vi "MSEncoder SubVI WfmCodeAccess PhaseScanII.vi"(6 "beta":ext, 8 "error in":errorcluster, 9 "Data in":T1, 11 "MSEncoder in":refnum<class "MSEncoder.lvclass">) -> (0 "error out":errorcluster, 1 "Scan time":dbl, 2 "mzTable":cluster{"t":dbl[], "mz":dbl[], "beta":dbl[]}, 3 "MSEncoder out":refnum<class "MSEncoder.lvclass">)   [LabVIEW 2018, in "MSEncoder.lvclass"]
uses:
  MSEncoder.lvclass
  MSEncoder.lvclass/MSEncoder.ctl
  WfmDataAccessor/WfmDataAccessor.lvclass
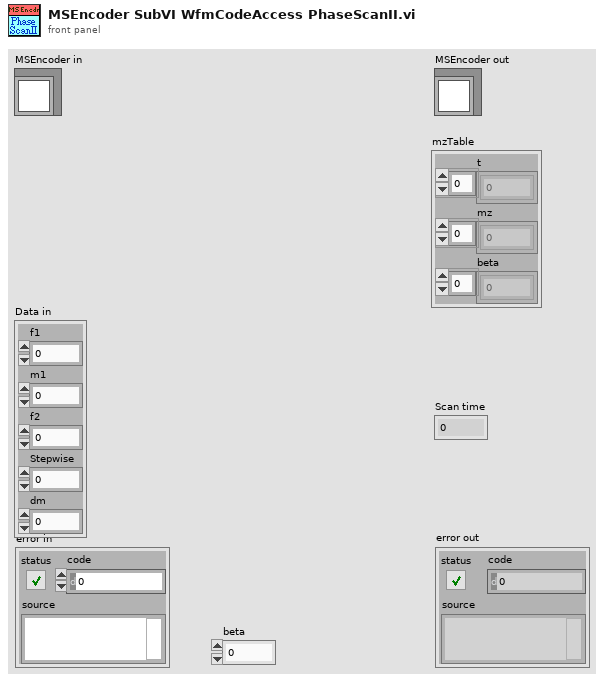
[diagram p1: front panel]
types:
  T1 = cluster{"f1":ext, "m1":ext, "f2":ext, "Stepwise":u32, "dm":ext}
  T2 = cluster{"Data in":cluster{"f1":ext, "m1":ext, "f2":ext, "Stepwise":u32, "dm":ext}, "CycDiff":u64[], "Ratio":u16[], "1/Decyc":u32, "Decyc":u32, string}
  T3 = cluster{"1/Decyc":u32, "Decyc":u64, "Actual Freq":dbl}
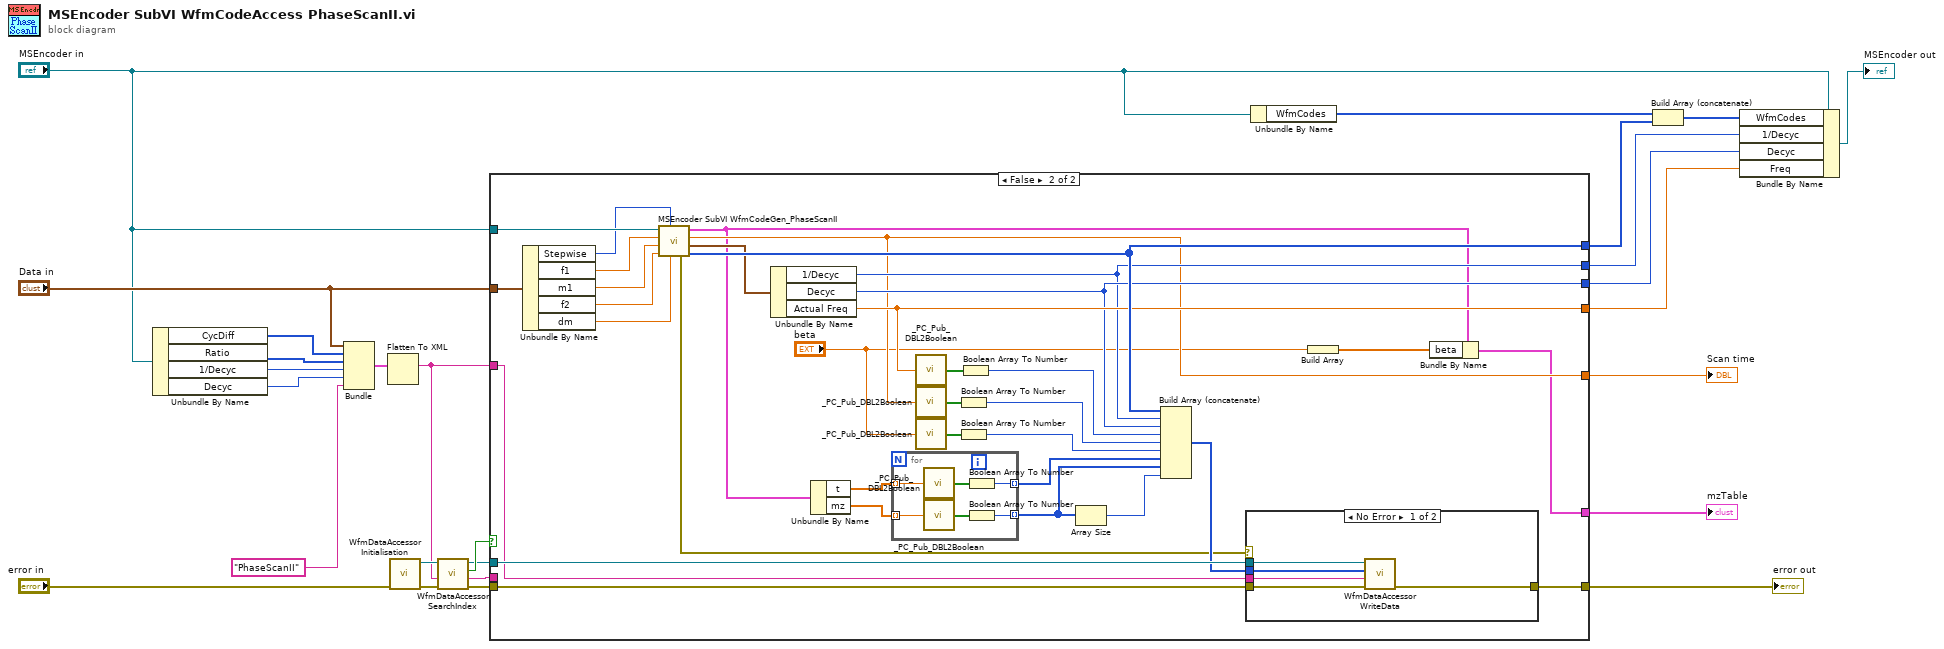
[diagram p0: block diagram]
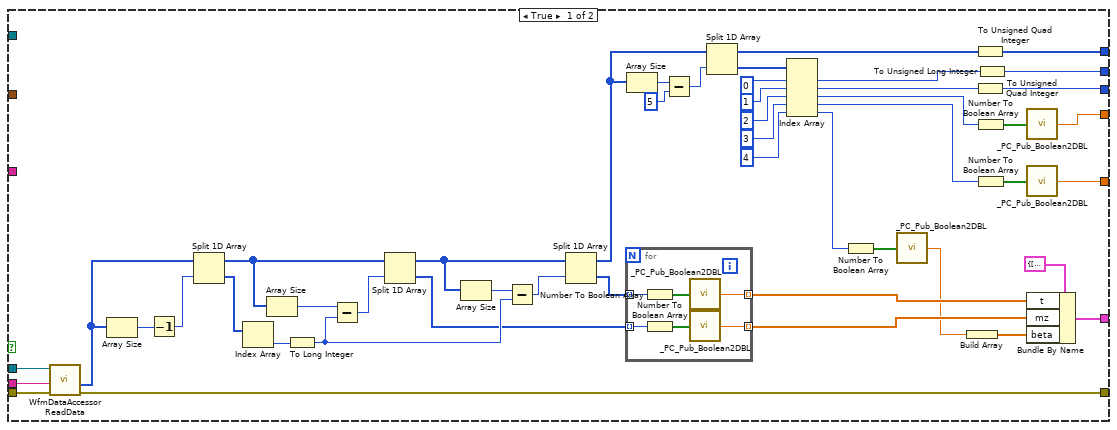
[diagram p2: hidden frame]
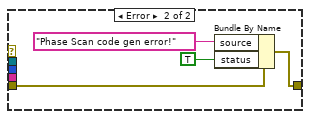
[diagram p3: hidden frame]
diagram:
  n1 = Unbundle By Name("MSEncoder in") -> ("CycDiff"=w21:u64[], "Ratio"=w22:u16[], "1/Decyc"=w23:u32, "Decyc"=w24:u32)
  n2 = Bundle("Data in"="Data in", "CycDiff"=w21, "Ratio"=w22, "1/Decyc"=w23, "Decyc"=w24, "PhaseScanII") -> (w20:T2)  [unwired: 1 in]
  n3 = Flatten To XML(anything=w20) -> (xml string=w13:string)
  n4 = call "WfmDataAccessor Initialisation.vi"("error in (no error)"="error in") -> ("error out"=w14:errorcluster, "WfmDataAccessor out"=w15:refnum<class "WfmDataAccessor.lvclass">)  [unwired: 9 in]
  n5 = call-dynamic "WfmDataAccessor SearchIndex.vi"("error in (no error)"=w14, "XML in"=w13, "WfmDataAccessor in"=w15) -> ("error out"=w10:errorcluster, "filename"=w9:string, "Found"=w12:bool, "WfmDataAccessor out"=w11:refnum<class "WfmDataAccessor.lvclass">)  [unwired: 5 in]
  n6 = case shown="False" w12 {
    tunnel: "MSEncoder in" -> [_ w106]
    tunnel: "Data in" -> [_ w107]
    tunnel: [w56 w97] -> w16
    tunnel: [w68 w104] -> w19
    tunnel: [w62 w95] -> w18
    tunnel: [w64 w96] -> w17
    tunnel: [w39 w108] -> w4
    tunnel: w13 -> [_ w109]
    tunnel: w11 -> [w61 w114]
    tunnel: w10 -> [w60 w110]
    tunnel: w9 -> [w59 _]
    tunnel: [w45 w82] -> w2
    tunnel: [w42 w90] -> w1
    frame True {
      n7 = call-dynamic "WfmDataAccessor ReadData.vi"("error in (no error)"=w60, "Filename"=w59, "WfmDataAccessor in"=w61) -> ("error out"=w39:errorcluster, "WfmData"=w53:u64[])  [unwired: 6 in, 1 out]
      n8 = Array Size(array=w53) -> (size(s)=w54:i32)
      n9 = Decrement(x=w54) -> (x-1=w55:i32)
      n10 = Split 1D Array(array=w53, index=w55) -> (first subarray=w40:u64[], second subarray=w52:u64[])
      n11 = Index Array(array=w52) -> (element=w50:u64)  [unwired: 1 in]
      n12 = Array Size(array=w40) -> (size(s)=w38:i32)
      n13 = To Long Integer(number=w50) -> (32bit integer=w37:i32)
      n14 = Subtract(x=w38, y=w37) -> (x-y=w36:i32)
      n15 = Split 1D Array(array=w40, index=w36) -> (first subarray=w34:u64[], second subarray=w32:u64[])
      n16 = Array Size(array=w34) -> (size(s)=w35:i32)
      n17 = Subtract(x=w35, y=w37) -> (x-y=w51:i32)
      n18 = Split 1D Array(array=w34, index=w51) -> (first subarray=w31:u64[], second subarray=w49:u64[])
      n19 = for {
        tunnel: w49 -> [w76] mode=indexing
        tunnel: [w78] -> w47 mode=indexing
        tunnel: [w77] -> w46 mode=indexing
        tunnel: w32 -> [w75] mode=indexing
        n20 = Number To Boolean Array(number=w76) -> (Boolean array=w80:bool[])
        n21 = Number To Boolean Array(number=w75) -> (Boolean array=w79:bool[])
        n22 = call "_PC_Pub_Boolean2DBL.vi"("Boolean array"=w80) -> ("DBL"=w78:dbl)
        n23 = call "_PC_Pub_Boolean2DBL.vi"("Boolean array"=w79) -> ("DBL"=w77:dbl)
      }
      n24 = Array Size(array=w31) -> (size(s)=w74:i32)
      n25 = Subtract(x=w74, y=5) -> (x-y=w72:i32)
      n26 = Split 1D Array(array=w31, index=w72) -> (first subarray=w69:u64[], second subarray=w71:u64[])
      n27 = Index Array(array=w71, index #1=0 ("index"), index #2=1 ("index"), index #3=2 ("index"), index #4=3 ("index"), index #5=4 ("index")) -> (element #1=w63:u64, element #2=w65:u64, element #3=w58:u64, element #4=w41:u64, element #5=w29:u64)
      n28 = Number To Boolean Array(number=w29) -> (Boolean array=w30:bool[])
      n29 = call "_PC_Pub_Boolean2DBL.vi"("Boolean array"=w30) -> ("DBL"=w28:dbl)
      n30 = Build Array(w28) -> (w27:dbl[])
      n31 = To Unsigned Quad Integer(1:w69) -> (0:w68:u64[])
      n32 = To Unsigned Quad Integer(1:w65) -> (0:w64:u64)
      n33 = Number To Boolean Array(number=w58) -> (Boolean array=w57:bool[])
      n34 = Number To Boolean Array(number=w41) -> (Boolean array=w43:bool[])
      n35 = To Unsigned Long Integer(number=w63) -> (unsigned 32bit integer=w62:u32)
      n36 = call "_PC_Pub_Boolean2DBL.vi"("Boolean array"=w57) -> ("DBL"=w56:dbl)
      n37 = call "_PC_Pub_Boolean2DBL.vi"("Boolean array"=w43) -> ("DBL"=w42:dbl)
      n38 = Bundle By Name(cluster=cluster{"t":dbl[], "mz":dbl[], "beta":dbl[]} {"t"=[], "mz"=[], "beta"=[]} ("mzTable"), "t"=w47, "mz"=w46, "beta"=w27) -> (w45:cluster{"t":dbl[], "mz":dbl[], "beta":dbl[]})
    }
    frame False {
      n39 = Unbundle By Name(w107) -> ("Stepwise"=w105:u32, "f1"=w100:ext, "m1"=w101:ext, "f2"=w102:ext, "dm"=w99:ext)
      n40 = call "MSEncoder SubVI WfmCodeGen_PhaseScanII.vi"("dm"=w99, "Stepwise"=w105, "f2"=w102, "m1"=w101, "f1"=w100, "MSEncoder.lvclass"=w106) -> ("WfmCode"=w104:u64[], "RF status"=w98:T3, "Scan time"=w90:dbl, "mzTable"=w81:cluster{"t":dbl[], "mz":dbl[], "beta":dbl[]}, "error out"=w103:errorcluster)  [unwired: 1 in]
      n41 = Unbundle By Name(w98) -> ("1/Decyc"=w95:u32, "Decyc"=w96:u64, "Actual Freq"=w97:dbl)
      n42 = Unbundle By Name(w81) -> ("t"=w92:dbl[], "mz"=w91:dbl[])
      n43 = for {
        tunnel: w92 -> [w119] mode=indexing
        tunnel: w91 -> [w117] mode=indexing
        tunnel: [w116] -> w87 mode=indexing
        tunnel: [w115] -> w86 mode=indexing
        n44 = call "_PC_Pub_DBL2Boolean.vi"("DBL"=w119) -> ("Boolean array"=w120:bool[])
        n45 = call "_PC_Pub_DBL2Boolean.vi"("DBL"=w117) -> ("Boolean array"=w118:bool[])
        n46 = Boolean Array To Number(Boolean array=w120) -> (number=w115:u64)
        n47 = Boolean Array To Number(Boolean array=w118) -> (number=w116:u64)
      }
      n48 = call "_PC_Pub_DBL2Boolean.vi"("DBL"=w97) -> ("Boolean array"=w113:bool[])
      n49 = call "_PC_Pub_DBL2Boolean.vi"("DBL"=w90) -> ("Boolean array"=w94:bool[])
      n50 = call "_PC_Pub_DBL2Boolean.vi"("DBL"="beta") -> ("Boolean array"=w88:bool[])
      n51 = Boolean Array To Number(Boolean array=w94) -> (number=w93:u64)
      n52 = Boolean Array To Number(Boolean array=w88) -> (number=w85:u64)
      n53 = Boolean Array To Number(Boolean array=w113) -> (number=w112:u64)
      n54 = Array Size(array=w87) -> (size(s)=w89:i32)
      n55 = Build Array (concatenate)(w104, w95, w96, w112, w93, w85, w86, w87, w89) -> (w111:u64[])
      n56 = case shown="No Error" w103 {
        tunnel: w114 -> [w125 _]
        tunnel: w111 -> [w124 _]
        tunnel: w110 -> [w123 w127]
        tunnel: w109 -> [w122 _]
        tunnel: [w121 w126] -> w108
        frame No Error {
          n57 = call-dynamic "WfmDataAccessor WriteData.vi"("error in (no error)"=w123, "XML"=w122, "WfmData"=w124, "WfmDataAccessor in"=w125) -> ("error out"=w121:errorcluster)  [unwired: 6 in, 1 out]
        }
        frame Error {
          n58 = Bundle By Name(cluster=w127, "source"="Phase Scan code gen error!", "status"=TRUE) -> (w126:errorcluster)
        }
      }
      n59 = Build Array("beta") -> (w83:ext[])
      n60 = Bundle By Name(cluster=w81, "beta"=w83) -> (w82:cluster{"t":dbl[], "mz":dbl[], "beta":dbl[]})
    }
  }
  "error out" <- w4
  "mzTable" <- w2
  "Scan time" <- w1
  n61 = Unbundle By Name("MSEncoder in") -> ("WfmCodes"=w26:u64[])
  n62 = Build Array (concatenate)(w26, w19) -> (w25:u64[])
  n63 = Bundle By Name(cluster="MSEncoder in", "WfmCodes"=w25, "1/Decyc"=w18, "Decyc"=w17, "Freq"=w16) -> (→"MSEncoder out":refnum<class "MSEncoder.lvclass">)
